vi "Send If Error In.vi"(8 "error in":errorcluster, 10 "Error Message Label (optional)":string, 11 "Send in":refnum<class "Send.lvclass">) -> (0 "Warning out":errorcluster, 3 "Send out":refnum<class "Send.lvclass">)   [LabVIEW 2011, in "Messenging.lvlib" / "Send.lvclass"]
uses:
  Send.lvclass
  ErrorMessage/ErrorMessage.lvclass
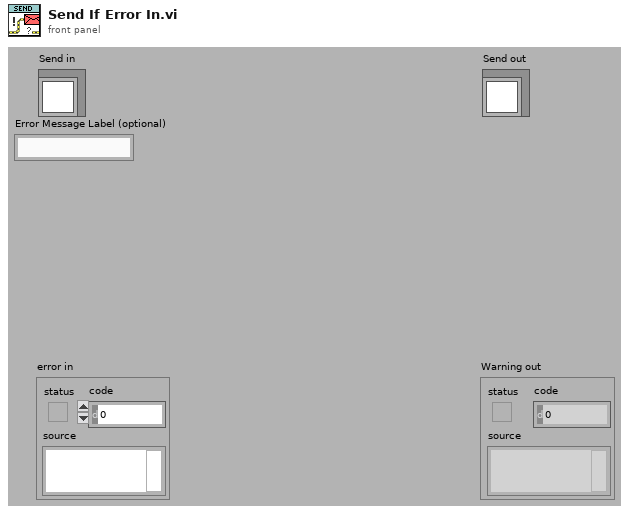
[diagram p1: front panel]
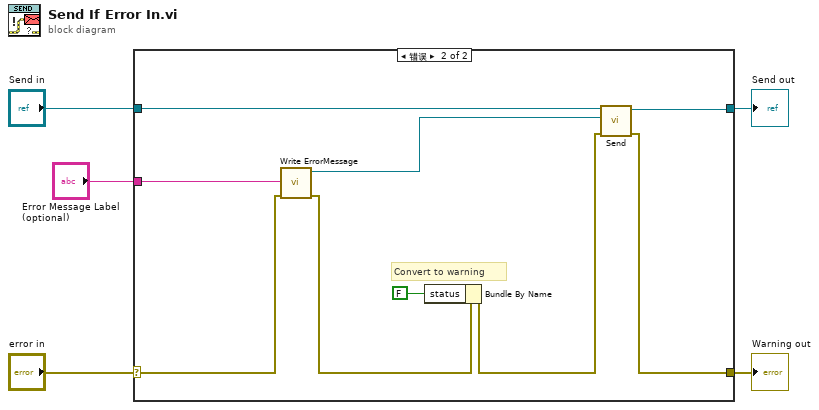
[diagram p0: block diagram]
diagram:
  n1 = case shown="错误" "error in" {
    selector: "error in" -> [w6 w12]
    tunnel: [w6 w9] -> w4
    tunnel: [w7 w15] -> w2
    tunnel: "Send in" -> [w7 w16]
    tunnel: "Error Message Label (optional)" -> [_ w8]
    frame No Error {
      # "Wire the error cluster across even in the \"No Error\"\ncase so that warnings get propagated."
    }
    frame Error {
      # "Convert to warning"
      n2 = call "Write ErrorMessage.vi"("error (to be sent)"=w12, "Label"=w8) -> ("error out"=w11:errorcluster, "Message"=w14:refnum<class "ErrorMessage.lvclass">)  [unwired: 1 in, 7 out]
      n3 = Bundle By Name(cluster=w11, "status"=FALSE) -> (w10:errorcluster)
      n4 = call-dynamic "Send.vi"("error in (no error)"=w10, "Message"=w14, "MSR Parent in"=w16) -> ("error out"=w9:errorcluster, "MSR Parent out"=w15:refnum<class "Send.lvclass">)  [unwired: 7 out]
    }
  }
  "Warning out" <- w4
  "Send out" <- w2
